vi "Send Image to HOST (SubVI).vi"(5 "Pixel Data":u64, 7 "Input Valid":bool) -> ()   [LabVIEW 2015]
uses:
  <vilib>/rvi/interface/RandomDataEmulation/niFpgaRandomDataHandleErrors.vi
  <vilib>/rvi/DataTransferAndStorage/Container/XNode/niFpgaContainer.xnode
  <vilib>/rvi/interface/RandomDataEmulation/nirviRandomDataFpgaReadWriteTemplate.vi
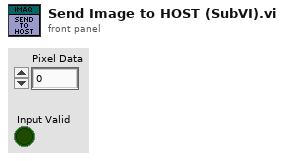
[diagram p1: front panel]
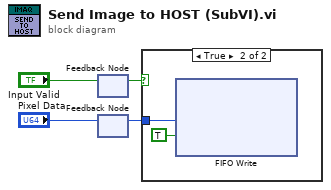
[diagram p0: block diagram]
diagram:
  n1 = feedback-in #1("Input Valid") -> ()
  n2 = feedback #1() -> (w2:bool)  [unwired: 1 in]
  n3 = feedback-in #2("Pixel Data") -> ()
  n4 = feedback #2() -> (w1:u64)  [unwired: 1 in]
  n5 = case shown="True" w2 {
    tunnel: w1 -> [_ w6]
    frame False {
    }
    frame True {
      n6 = xnode ("FIFO Write")("Element"=w6, "Input Valid"=TRUE) -> ()  [unwired: 1 in, 2 out]
    }
  }
